vi "Simulated Data.vi"(0 "Polarity":bool) -> (1 "Cluster":T2 {"Frequency (MHz)" format="%.2f"; "Amplitude (Vrms)" format="%.2p"}, 2 "Amplitude Spectrum":T1 {"dB Spectrum (Hann)" format="%.2f"; "df" format="%.2f"; "f0" format="%.2f"})   [LabVIEW 2012]
uses:
  <vilib>/Waveform/WDTOps.llb/WDT Number of Waveform Samples DBL.vi
  <vilib>/measure/madcrms.llb/Basic Averaged DC-RMS for 1 Chan.vi
  <vilib>/measure/NI_MABase.lvlib
  <vilib>/measure/NI_MAPro.lvlib
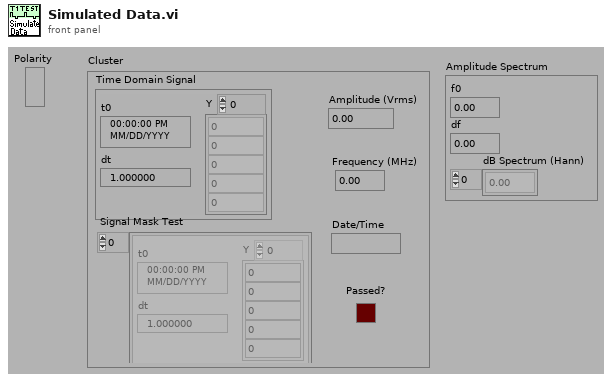
[diagram p1: front panel]
types:
  T1 = cluster{"f0":dbl, "df":dbl, "dB Spectrum (Hann)":dbl[]}
  T2 = cluster{"Time Domain Signal":waveform(dbl), "Signal Mask Test":waveform(dbl)[], "Amplitude (Vrms)":dbl, "Frequency (MHz)":dbl, "Date/Time":string, "Passed?":bool}
  T3 = enum16{"Rectangular (none)", "Hanning", "Low side lobe"}
  T4 = cluster{"waveform out":waveform(dbl), "output values":waveform(dbl)[], "RMS value":dbl, dbl, string, "test passed?":bool}
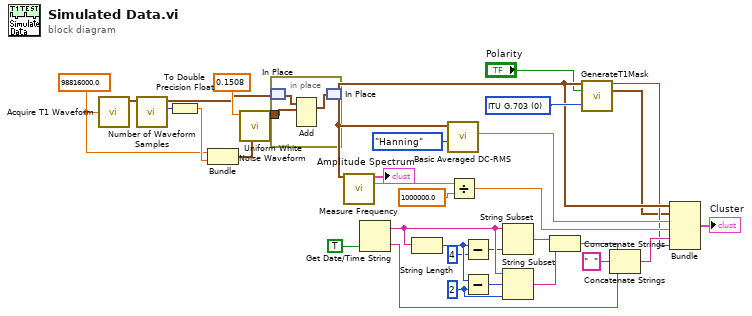
[diagram p0: block diagram]
diagram:
  w16 = 98816000.0 ("sampling frequency")
  w21 = u16 0 items=["ITU G.703", "EIA/TIA 547"] ("Standard")
  w28 = 2 ("y")
  n1 = call "Acquire T1 Waveform.vi"("sampling frequency"=w16) -> ("Waveform"=w13:waveform(dbl))  [unwired: 13 in, 1 out]
  n2 = call-poly <vilib>:"Number of Waveform Samples.vi"("waveform in"=w13) -> ("number of samples"=w17:i32, "waveform out"=w14:waveform(dbl))  [unwired: 8 in, 1 out]
  n3 = To Double Precision Float(number=w17) -> (double precision float=w19:dbl)
  n4 = Bundle("sampling frequency"=w16, w19) -> (w18:cluster{"sampling frequency":dbl, dbl})  [unwired: 1 in]
  n5 = call <vilib>:"Uniform White Noise Waveform.vi"("sampling info"=w18, "amplitude"=0.1508) -> ("signal out"=w15:waveform(dbl))  [unwired: 8 in, 1 out]
  n6 = in-place {
    in-place-border: w15 -> [w36]
    n7 = in-place-match #1(w14) -> (w35:waveform(dbl))
    n8 = Add ("Add Waveforms.vi")(1:w36, 2:w35) -> (0:w34:waveform(dbl))  [unwired: 1 in, 1 out]
    n9 = in-place-match #1(w34) -> (w6:waveform(dbl))
  }
  n10 = call "Measure Frequency.vi"("Waveform"=w6) -> ("exported spectrum (dB)"=→"Amplitude Spectrum":T1, "frequency"=w12:dbl)  [unwired: 11 in, 2 out]
  n11 = Get Date/Time String(want seconds? (F)=TRUE) -> (date string=w31:string, time string=w33:string)  [unwired: 2 in]
  n12 = String Length(string=w31) -> (length=w25:i32)
  n13 = call-poly <vilib>:"Basic Averaged DC-RMS.vi"("window"=T3."Hanning", "signal in"=w6) -> ("RMS value"=w7:dbl)  [unwired: 6 in, 3 out]
  n14 = Divide(x=w12, y=1000000.0 ("Sampling Frequency")) -> (x/y=w8:dbl)
  n15 = Subtract(x=w25, y=4) -> (x-y=w26:i32)
  n16 = Subtract(x=w25, y=w28) -> (x-y=w27:i32)
  n17 = String Subset(string=w31, length (rest)=w26) -> (substring=w29:string)  [unwired: 1 in]
  n18 = String Subset(string=w31, offset (0)=w27, length (rest)=w28) -> (substring=w30:string)
  n19 = Concatenate Strings(w29, w30) -> (w32:string)
  n20 = call "GenerateT1Mask.vi"("Waveform"=w6, "Polarity"="Polarity", "Mask Selector"=w21) -> ("test passed?"=w3:bool, "output values"=w2:waveform(dbl)[])  [unwired: 10 in, 1 out]
  n21 = Concatenate Strings(w32, "  " ("Substring"), w33) -> (w9:string)
  n22 = Bundle("waveform out"=w6, "output values"=w2, "RMS value"=w7, w8, w9, "test passed?"=w3) -> (→"Cluster":T4)  [unwired: 1 in]
